vi "pp2_DAQclear.vi"(8 "error in (no error)":errorcluster, 11 "Daq config in":T1={"Sound AO"="Dev2/ao0", "Shock intesity AO"="Dev1/ao1", "Code_LED DO"="Dev1/port1:2", "Switch DI"="Dev1/port0/line0:1", "Webcam"="cam0", "Sound AO task"="", "Sound card task"=0, "Shock intensity AO task"="", "Code_LED DO task"="", "Switch DI task"="", "AO <=> Sound card"=FALSE, "Sound card"=0, "sample rate"=8000.0, "Variable shock"=FALSE, "Webcam on"=FALSE, "Tone gate PFI"="/Dev1/PFI1", "Waveform memo"={"t0"=timestamp(0 s since 1904-01-01), "dt"=1.0, "Y"=[]}, "First time"=FALSE} {"sample rate" min=8000.0; "Sound card task" format="%.0x"}) -> (0 "error out":errorcluster, 3 "Daq config out":T1={"Sound AO"="Dev2/ao0", "Shock intesity AO"="Dev1/ao1", "Code_LED DO"="Dev1/port1:2", "Switch DI"="Dev1/port0/line0:1", "Webcam"="cam0", "Sound AO task"="", "Sound card task"=0, "Shock intensity AO task"="", "Code_LED DO task"="", "Switch DI task"="", "AO <=> Sound card"=FALSE, "Sound card"=0, "sample rate"=8000.0, "Variable shock"=FALSE, "Webcam on"=FALSE, "Tone gate PFI"="/Dev1/PFI1", "Waveform memo"={"t0"=timestamp(0 s since 1904-01-01), "dt"=1.0, "Y"=[]}, "First time"=FALSE} {"sample rate" min=8000.0; "Sound card task" format="%.0x"})   [LabVIEW 2013]
uses:
  pp2_CTL_DaqConfig.ctl
  <vilib>/userdefined/High Color/IMAQdx.ctl
  <vilib>/sound2/lvsound2.llb/Sound Output Task ID.ctl
  <resource>/objmgr/daqmx.rc
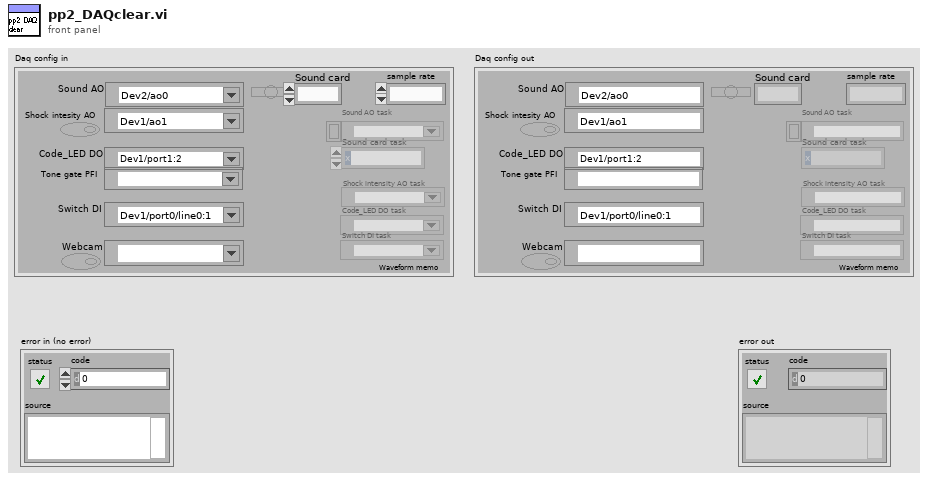
[diagram p1: front panel]
types:
  T1 = typedef "pp2_CTL_DaqConfig.ctl" = cluster{"Sound AO":tag, "Shock intesity AO":tag, "Code_LED DO":tag, "Switch DI":tag, "Webcam":T2, "Sound AO task":refnum<k21>, "Sound card task":T3, "Shock intensity AO task":refnum<k21>, "Code_LED DO task":refnum<k21>, "Switch DI task":refnum<k21>, "AO <=> Sound card":bool, "Sound card":u32, "sample rate":dbl, "Variable shock":bool, "Webcam on":bool, "Tone gate PFI":tag, "Waveform memo":waveform(dbl), "First time":bool}
  T2 = typedef "IMAQdx.ctl" = refnum<k21>
  T3 = typedef "Sound Output Task ID.ctl" = u32
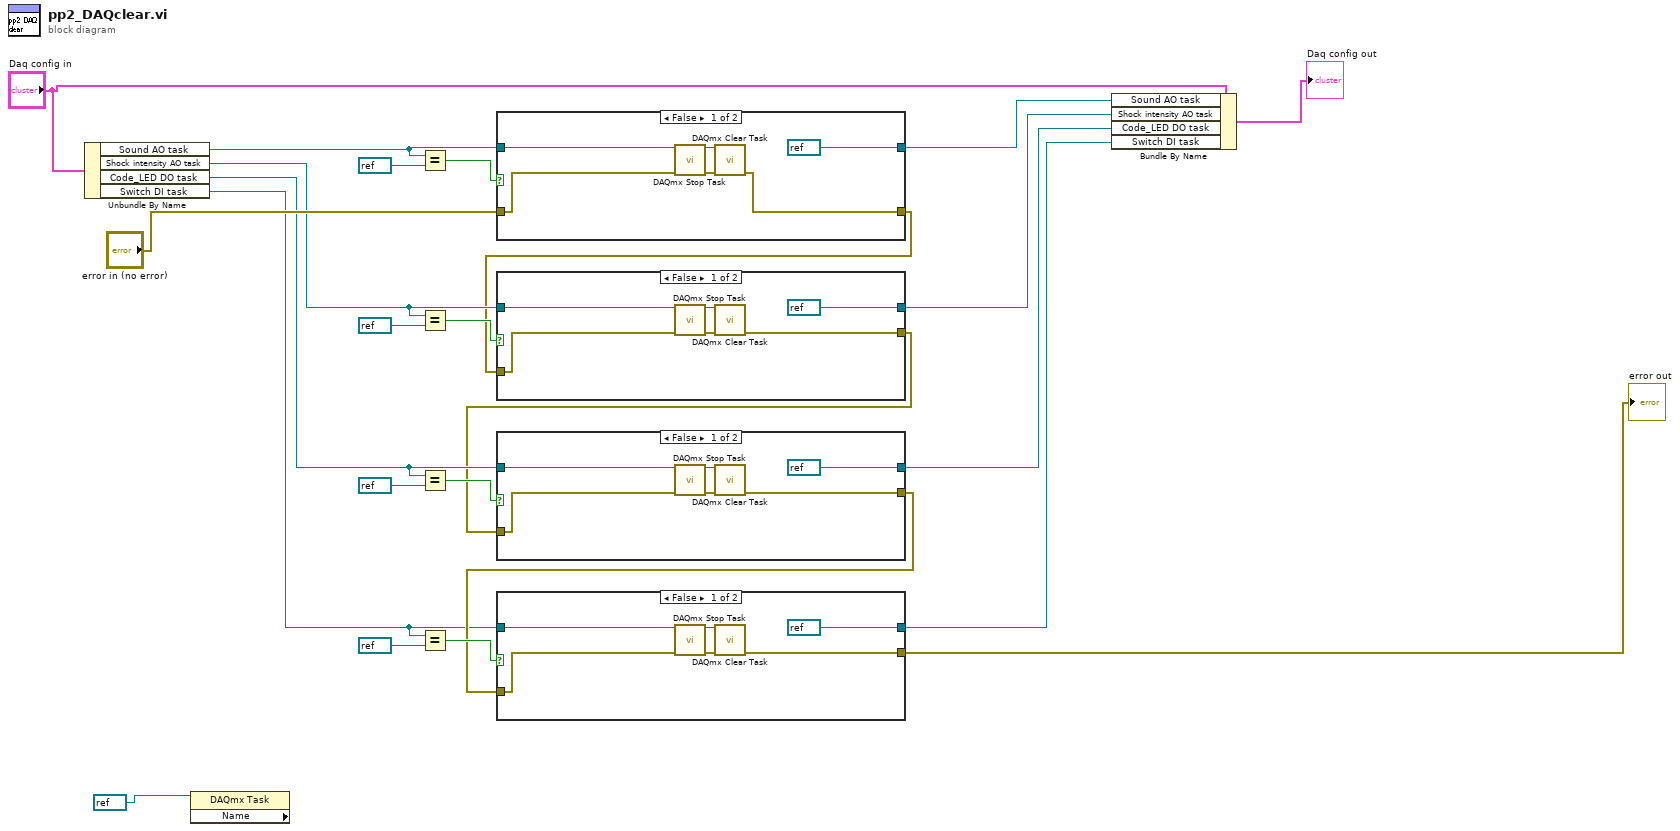
[diagram p0: block diagram]
diagram:
  n1 = Unbundle By Name("Daq config in") -> ("Sound AO task"=w13:refnum<k21>, "Shock intensity AO task"=w8:refnum<k21>, "Code_LED DO task"=w7:refnum<k21>, "Switch DI task"=w2:refnum<k21>)
  n2 = property class="DAQmx Task" props=["Name"](reference=refnum<k21> refnum ("y")) -> ()  [unwired: 1 in, 3 out]
  n3 = Equal?(x=w13, y=refnum<k21> refnum) -> (x = y?=w23:bool)
  n4 = Equal?(x=w8, y=refnum<k21> refnum) -> (x = y?=w18:bool)
  n5 = Equal?(x=w7, y=refnum<k21> refnum) -> (x = y?=w16:bool)
  n6 = Equal?(x=w2, y=refnum<k21> refnum) -> (x = y?=w14:bool)
  n7 = case shown="False" w23 {
    tunnel: w13 -> [w28 w32]
    tunnel: [refnum<k21> refnum ("NULL") w32] -> w22
    tunnel: "error in (no error)" -> [w27 w31]
    tunnel: [w25 w31] -> w6
    frame False {
      n8 = call <vilib>:"DAQmx Stop Task.vi"("task/channels in"=w28, "error in"=w27) -> ("task out"=w30:refnum<k21>, "error out"=w29:errorcluster)  [unwired: 12 in]
      n9 = call <vilib>:"DAQmx Clear Task.vi"("task in"=w30, "error in"=w29) -> ("error out"=w25:errorcluster)  [unwired: 13 in]
    }
    frame True {
    }
  }
  n10 = case shown="False" w18 {
    tunnel: w8 -> [w36 w40]
    tunnel: [refnum<k21> refnum ("NULL") w40] -> w11
    tunnel: w6 -> [w35 w39]
    tunnel: [w33 w39] -> w5
    frame False {
      n11 = call <vilib>:"DAQmx Stop Task.vi"("task/channels in"=w36, "error in"=w35) -> ("task out"=w38:refnum<k21>, "error out"=w37:errorcluster)  [unwired: 12 in]
      n12 = call <vilib>:"DAQmx Clear Task.vi"("task in"=w38, "error in"=w37) -> ("error out"=w33:errorcluster)  [unwired: 13 in]
    }
    frame True {
    }
  }
  n13 = case shown="False" w16 {
    tunnel: w7 -> [w44 w48]
    tunnel: [refnum<k21> refnum ("NULL") w48] -> w10
    tunnel: w5 -> [w43 w47]
    tunnel: [w41 w47] -> w4
    frame False {
      n14 = call <vilib>:"DAQmx Stop Task.vi"("task/channels in"=w44, "error in"=w43) -> ("task out"=w46:refnum<k21>, "error out"=w45:errorcluster)  [unwired: 12 in]
      n15 = call <vilib>:"DAQmx Clear Task.vi"("task in"=w46, "error in"=w45) -> ("error out"=w41:errorcluster)  [unwired: 13 in]
    }
    frame True {
    }
  }
  n16 = case shown="False" w14 {
    tunnel: w2 -> [w52 w56]
    tunnel: [refnum<k21> refnum ("NULL") w56] -> w9
    tunnel: w4 -> [w51 w55]
    tunnel: [w49 w55] -> w3
    frame False {
      n17 = call <vilib>:"DAQmx Stop Task.vi"("task/channels in"=w52, "error in"=w51) -> ("task out"=w54:refnum<k21>, "error out"=w53:errorcluster)  [unwired: 12 in]
      n18 = call <vilib>:"DAQmx Clear Task.vi"("task in"=w54, "error in"=w53) -> ("error out"=w49:errorcluster)  [unwired: 13 in]
    }
    frame True {
    }
  }
  "error out" <- w3
  n19 = Bundle By Name(cluster="Daq config in", "Sound AO task"=w22, "Shock intensity AO task"=w11, "Code_LED DO task"=w10, "Switch DI task"=w9) -> (→"Daq config out":T1)
